vi "主程序.vi"() -> ()   [LabVIEW 2013]
doc: "该模板用于创建生产者／消费者模式的应用程序，以事件驱动的方式，生成队列中的项。如需通过响应事件实现代码的异步执行，同时不影响用户界面的响应速度，可考虑用该模式替代“用户界面事件处理器”模式。"
uses:
  <vilib>/Instr/_visa.llb/VISA Configure Serial Port (Instr).vi
panel:
  out "8位验证":string
  out "17位验证":string
  in  "参数保存":bool
  in  "执行次数":i32=3
  in  "减速（Max=65535）":i32=550 max=65535
  in  "加速（Max=65535）":i32=550 max=65535
  in  "行进距离（Max=16777214）":i32=25500 max=16777214
  out "低位":string
  out "高位":string
  out "运行速度（256-65535）":i32
  in  "位置控制模式":bool
  in  "模式选择":string(combo)="\u0000"
  in  "速度增减幅度":i32(ring)=1 items=["1"=1, "10"=10, "20"=20, "50"=50, "100"=100, "200"=200, "500"=500, "1000"=1000, "2000"=2000, "5000"=5000, "10000"=10000]
  in  "速度-":bool
  in  "速度+":bool
  in  "运行速度（256-65535）":i32=63500 min=256 max=65535
  in  "停止运行":bool
  in  "负向运行":bool
  in  "正向运行":bool
  in  "停止":bool
  in  "端口开关":bool
  in  "端口选择":refnum<visa-resource-name>
  # "步进电机控制系统"
  # "请关闭端口开关后再停止程序！"
  # "设置好相关参数后点击参数保存"
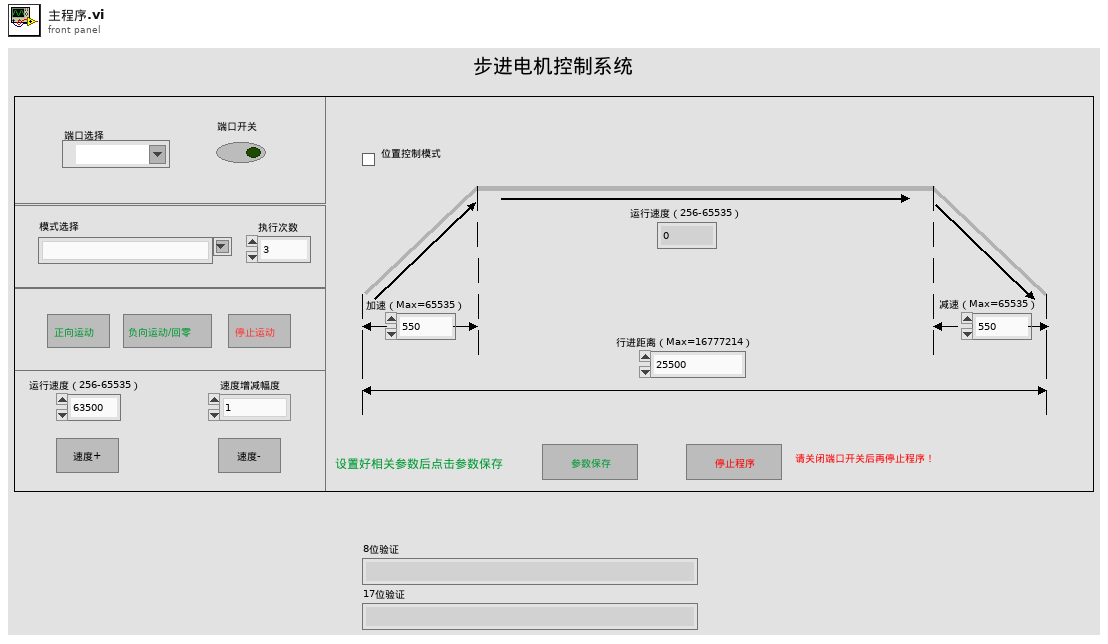
[diagram p1: front panel]
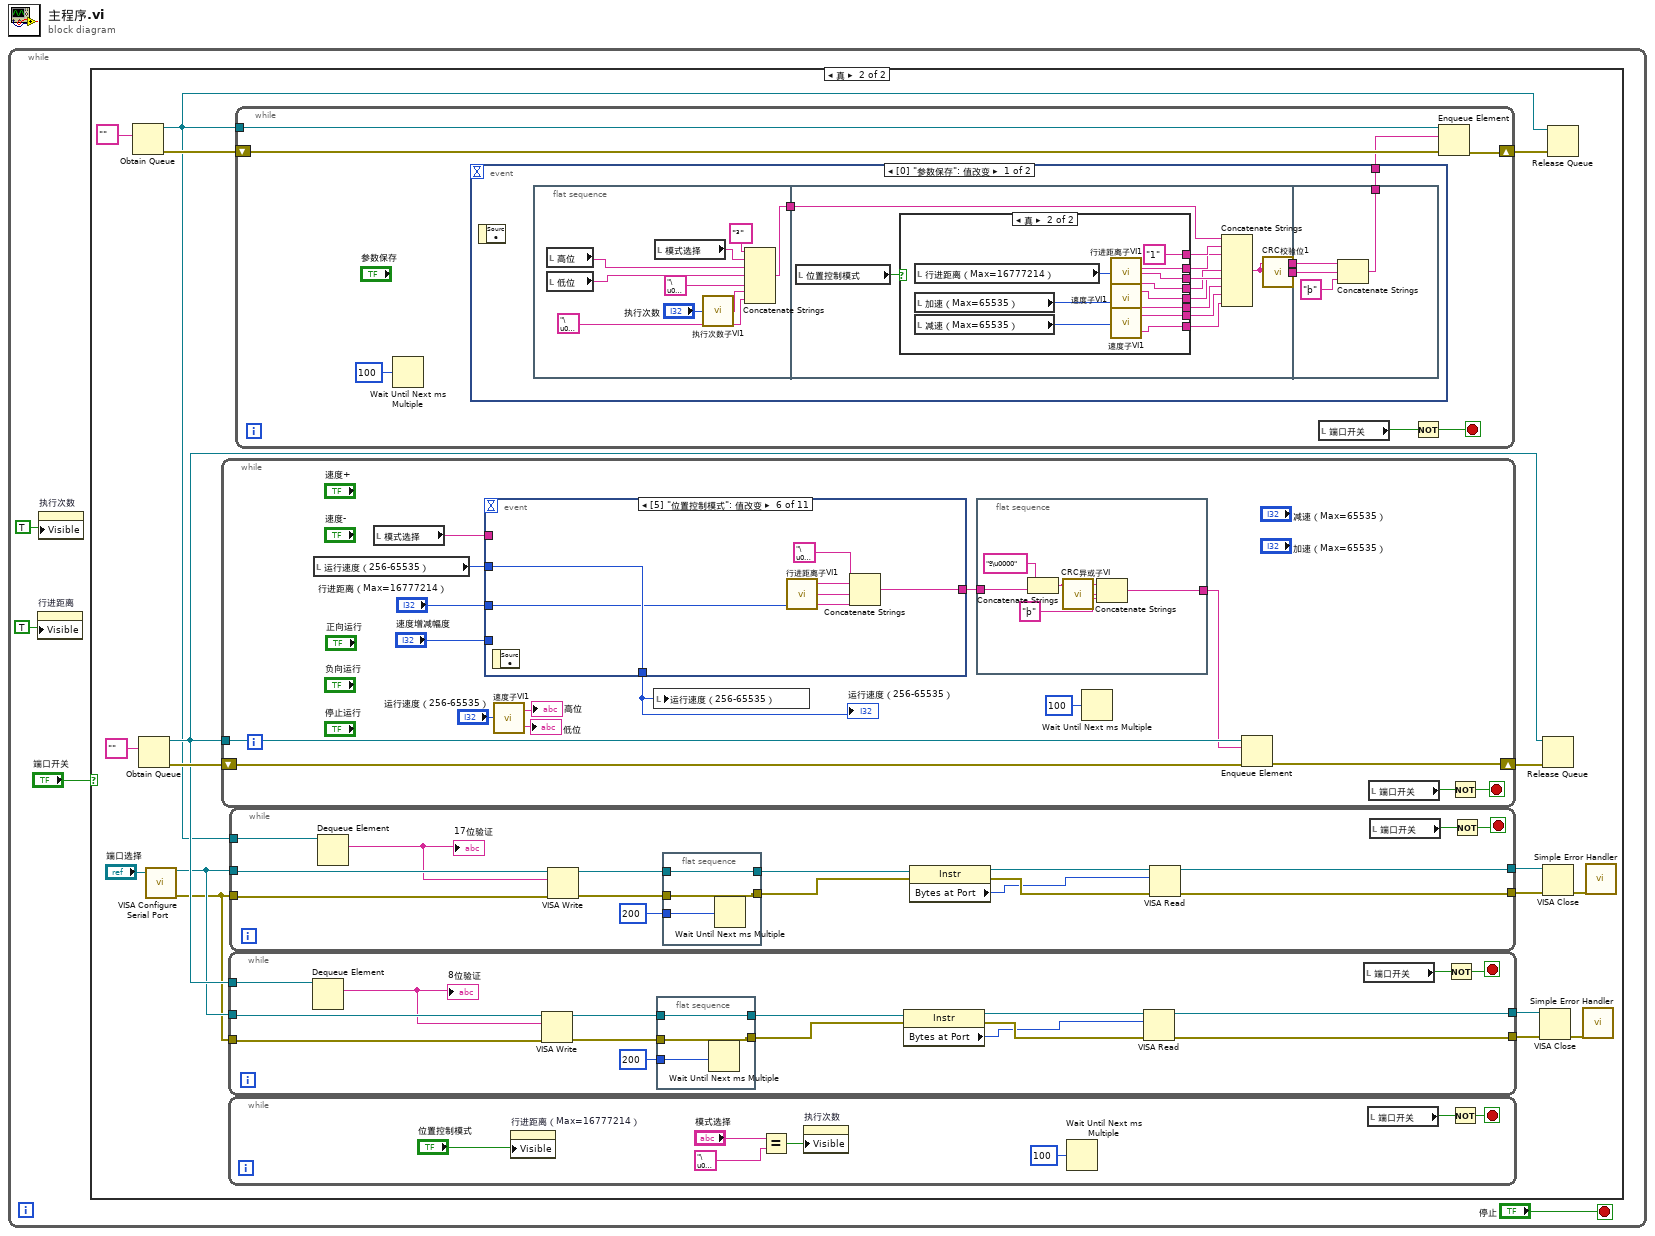
[diagram p0: block diagram]
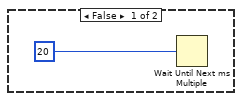
[diagram p2: hidden frame]
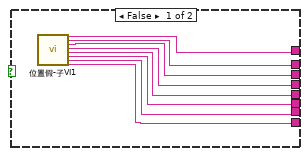
[diagram p3: hidden frame]
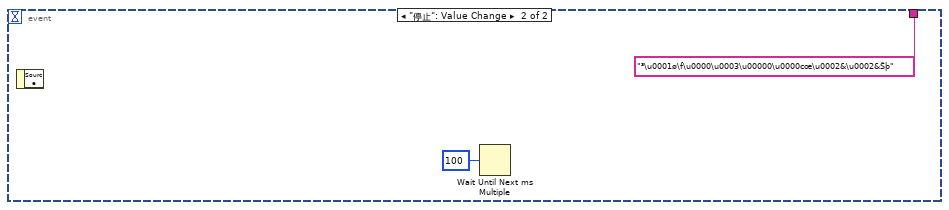
[diagram p4: hidden frame]
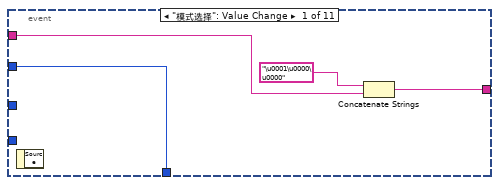
[diagram p5: hidden frame]
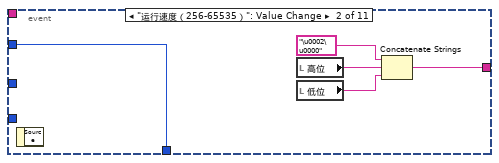
[diagram p6: hidden frame]
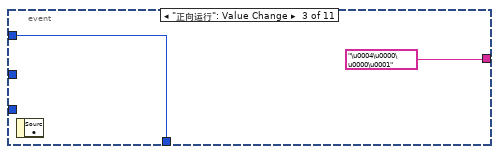
[diagram p7: hidden frame]
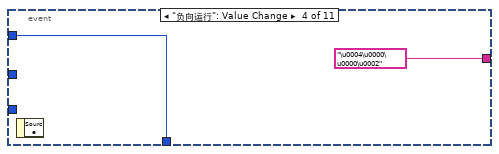
[diagram p8: hidden frame]
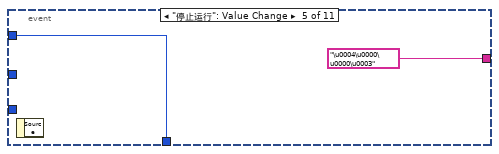
[diagram p9: hidden frame]
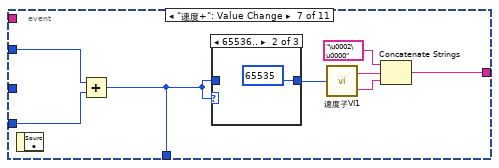
[diagram p10: hidden frame]
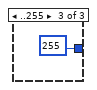
[diagram p12: hidden frame]
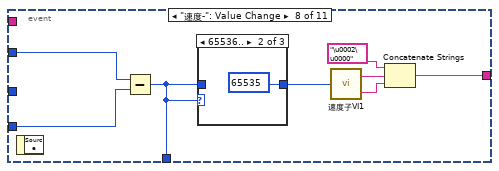
[diagram p13: hidden frame]
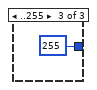
[diagram p15: hidden frame]
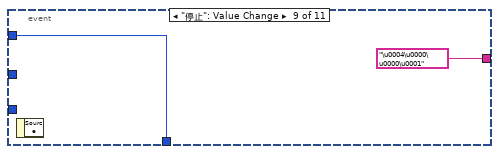
[diagram p16: hidden frame]
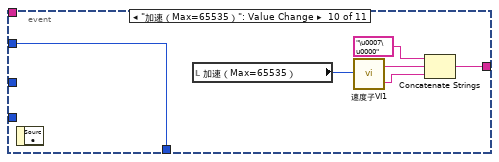
[diagram p17: hidden frame]
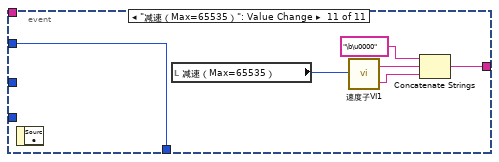
[diagram p18: hidden frame]
diagram:
  n1 = while {
    stop <- "停止" stop-if-true
    n2 = property on="行进距离" class="DigNum (严格)"("Visible"=TRUE) -> ()  [unwired: 2 in, 2 out]
    n3 = property on="执行次数" class="DigNum (严格)"("Visible"=TRUE) -> ()  [unwired: 2 in, 2 out]
    n4 = case shown="真" "端口开关" {
      frame False {
        n5 = Wait Until Next ms Multiple(millisecond multiple=u32 20 ("毫秒计时值")) -> ()  [unwired: 1 out]
      }
      frame True {
        n6 = Obtain Queue(element data type="") -> (queue out=w6:refnum<queue>, error out=w15:errorcluster)  [unwired: 4 in, 1 out]
        n7 = Obtain Queue(element data type="") -> (queue out=w12:refnum<queue>, error out=w22:errorcluster)  [unwired: 4 in, 1 out]
        n8 = call-poly "VISA Configure Serial Port"("VISA resource name"="端口选择") -> ("VISA resource name out"=w11:refnum<visa-resource-name>, "error out"=w10:errorcluster)  [unwired: 13 in]
        n9 = while {
          shift-right: [w139] -> w21
          shift-left: w22 -> [w140]
          tunnel: w12 -> [w138]
          stop <- w130 stop-if-true
          n10 = local read "运行速度（256-65535）"() -> (w129:i32)
          n11 = local read "模式选择"() -> (w126:string)
          n12 = event shown="[5] \"位置控制模式\": 值改变" {
            selector: _ -> [_ _ _ _ _ _ _ _ _ _ _]
            dyn-events: _ -> [_ _ _ _ _ _ _ _ _ _ _]
            timeout: _ -> [_ _ _ _ _ _ _ _ _ _ _]
            tunnel: [w149 w152 "\u0004\u0000\u0000\u0001" "\u0004\u0000\u0000\u0002" "\u0004\u0000\u0000\u0003" w164 w173 w184 "\u0004\u0000\u0000\u0001" w194 w200] -> w134
            tunnel: [w148 w151 w156 w158 w160 w163 w170 w182 w191 w193 w199] -> w133
            tunnel: w129 -> [w148 w151 w156 w158 w160 w163 w171 w181 w191 w193 w199]
            tunnel: "速度增减幅度" -> [_ _ _ _ _ _ w169 w180 _ _ _]
            tunnel: w126 -> [w147 _ _ _ _ _ _ _ _ _ _]
            tunnel: "行进距离（Max=16777214）" -> [_ _ _ _ _ w162 _ _ _ _ _]
            event "模式选择": Value Change {
              n13 = event-data() -> ()  [unwired: 1 in, 1 out]
              n14 = Concatenate Strings("\u0001\u0000\u0000", w147) -> (w149:string)
            }
            event "运行速度（256-65535）": Value Change {
              n15 = event-data() -> ()  [unwired: 1 in, 1 out]
              n16 = local read "高位"() -> (w154:string)
              n17 = local read "低位"() -> (w153:string)
              n18 = Concatenate Strings("\u0002\u0000", w154, w153) -> (w152:string)
            }
            event "正向运行": Value Change {
              n19 = event-data() -> ()  [unwired: 1 in, 1 out]
            }
            event "负向运行": Value Change {
              n20 = event-data() -> ()  [unwired: 1 in, 1 out]
            }
            event "停止运行": Value Change {
              n21 = event-data() -> ()  [unwired: 1 in, 1 out]
            }
            event "位置控制模式": Value Change {
              n22 = event-data() -> ()  [unwired: 1 in, 1 out]
              n23 = call "行进距离子VI1.vi"("脉冲输入端"=w162) -> ("行进脉冲总数高位"=w167:string, "行进脉冲总数中位"=w166:string, "行进脉冲总数低位"=w165:string)
              n24 = Concatenate Strings("\u0006", w167, w166, w165) -> (w164:string)
            }
            event "速度+": Value Change {
              n25 = event-data() -> ()  [unwired: 1 in, 1 out]
              n26 = Add(x=w171, y=w169) -> (x+y=w170:i32)
              n27 = case shown="65536.." w170 {
                tunnel: w170 -> [w177 _ _]
                tunnel: [w177 65535 255] -> w172
                frame 256..65535 {
                }
                frame 65536.. {
                }
                frame ..255 {
                }
              }
              n28 = call "速度子VI1.vi"("脉冲数"=w172) -> ("分频基数高位"=w175:string, "分频基数低位"=w174:string)
              n29 = Concatenate Strings("\u0002\u0000", w175, w174) -> (w173:string)
            }
            event "速度-": Value Change {
              n30 = event-data() -> ()  [unwired: 1 in, 1 out]
              n31 = Subtract(x=w181, y=w180) -> (x-y=w182:i32)
              n32 = case shown="65536.." w182 {
                tunnel: w182 -> [w188 _ _]
                tunnel: [w188 65535 255] -> w183
                frame 256..65535 {
                }
                frame 65536.. {
                }
                frame ..255 {
                }
              }
              n33 = call "速度子VI1.vi"("脉冲数"=w183) -> ("分频基数高位"=w186:string, "分频基数低位"=w185:string)
              n34 = Concatenate Strings("\u0002\u0000", w186, w185) -> (w184:string)
            }
            event "停止": Value Change {
              n35 = event-data() -> ()  [unwired: 1 in, 1 out]
            }
            event "加速（Max=65535）": Value Change {
              n36 = event-data() -> ()  [unwired: 1 in, 1 out]
              n37 = local read "加速（Max=65535）"() -> (w198:i32)
              n38 = call "速度子VI1.vi"("脉冲数"=w198) -> ("分频基数高位"=w196:string, "分频基数低位"=w195:string)
              n39 = Concatenate Strings("\u0007\u0000", w196, w195) -> (w194:string)
            }
            event "减速（Max=65535）": Value Change {
              n40 = event-data() -> ()  [unwired: 1 in, 1 out]
              n41 = local read "减速（Max=65535）"() -> (w204:i32)
              n42 = call "速度子VI1.vi"("脉冲数"=w204) -> ("分频基数高位"=w202:string, "分频基数低位"=w201:string)
              n43 = Concatenate Strings("\b\u0000", w202, w201) -> (w200:string)
            }
          }
          "运行速度（256-65535）" <- w133
          n44 = call "速度子VI1.vi"("脉冲数"="运行速度（256-65535）") -> ("分频基数高位"=→"高位":string, "分频基数低位"=→"低位":string)
          n45 = local write "运行速度（256-65535）"(w133) -> ()
          n46 = flat-sequence {
            tunnel: w134 -> [w145]
            tunnel: [w141] -> w127
            frame #0 {
              n47 = Concatenate Strings("º\u0000", w145) -> (w144:string)
              n48 = call "CRC异或子VI.vi"("输入"=w144) -> ("输出"=w143:string)
              n49 = Concatenate Strings(w144, w143, "þ") -> (w141:string)
            }
          }
          n50 = Wait Until Next ms Multiple(millisecond multiple=u32 100 ("毫秒倍数")) -> ()  [unwired: 1 out]
          n51 = Enqueue Element(queue=w138, element=w127, error in (no error)=w140) -> (error out=w139:errorcluster)  [unwired: 1 in, 2 out]
          n52 = local read "端口开关"() -> (w131:bool)
          n53 = Not(x=w131) -> (.not. x?=w130:bool)
        }
        n54 = while {
          tunnel: w10 -> [w26]
          tunnel: w11 -> [w27]
          tunnel: [w32] -> w7
          tunnel: [w31] -> w8
          tunnel: w12 -> [w28]
          stop <- w29 stop-if-true
          n55 = Dequeue Element(queue=w28) -> (element=w24:string)  [unwired: 2 in, 3 out]
          "8位验证" <- w24
          n56 = VISA Write(VISA resource name=w27, write buffer=w24, error in (no error)=w26) -> (VISA resource name out=w38:refnum<visa-resource-name>, error out=w37:errorcluster)  [unwired: 1 out]
          n57 = flat-sequence {
            tunnel: w38 -> [w41]
            tunnel: w37 -> [w40]
            tunnel: [w41] -> w36
            tunnel: [w40] -> w34
            tunnel: u32 200 ("等待时间（毫秒）") -> [w39]
            frame #0 {
              n58 = Wait Until Next ms Multiple(millisecond multiple=w39) -> ()  [unwired: 1 out]
            }
          }
          n59 = property class="Instr"(reference=w36, error in=w34) -> (reference out=w35:refnum<visa-resource-name>, error out=w33:errorcluster, "Bytes at Port"=w25:u32)
          n60 = VISA Read(VISA resource name=w35, byte count=w25, error in (no error)=w33) -> (VISA resource name out=w32:refnum<visa-resource-name>, error out=w31:errorcluster)  [unwired: 2 out]
          n61 = local read "端口开关"() -> (w30:bool)
          n62 = Not(x=w30) -> (.not. x?=w29:bool)
        }
        n63 = while {
          stop <- w103 stop-if-true
          n64 = property on="行进距离（Max=16777214）" class="DigNum (严格)"("Visible"="位置控制模式") -> ()  [unwired: 2 in, 2 out]
          n65 = Equal?(x="模式选择", y="\u0004") -> (x = y?=w99:bool)
          n66 = property on="执行次数" class="DigNum (严格)"("Visible"=w99) -> ()  [unwired: 2 in, 2 out]
          n67 = Wait Until Next ms Multiple(millisecond multiple=u32 100 ("等待时间（毫秒）")) -> ()  [unwired: 1 out]
          n68 = local read "端口开关"() -> (w104:bool)
          n69 = Not(x=w104) -> (.not. x?=w103:bool)
        }
        n70 = while {
          tunnel: w10 -> [w109]
          tunnel: w11 -> [w110]
          tunnel: [w115] -> w19
          tunnel: [w114] -> w18
          tunnel: w6 -> [w111]
          stop <- w112 stop-if-true
          n71 = Dequeue Element(queue=w111) -> (element=w107:string)  [unwired: 2 in, 3 out]
          "17位验证" <- w107
          n72 = VISA Write(VISA resource name=w110, write buffer=w107, error in (no error)=w109) -> (VISA resource name out=w121:refnum<visa-resource-name>, error out=w120:errorcluster)  [unwired: 1 out]
          n73 = flat-sequence {
            tunnel: w121 -> [w124]
            tunnel: w120 -> [w123]
            tunnel: [w124] -> w119
            tunnel: [w123] -> w117
            tunnel: u32 200 ("等待时间（毫秒）") -> [w122]
            frame #0 {
              n74 = Wait Until Next ms Multiple(millisecond multiple=w122) -> ()  [unwired: 1 out]
            }
          }
          n75 = property class="Instr"(reference=w119, error in=w117) -> (reference out=w118:refnum<visa-resource-name>, error out=w116:errorcluster, "Bytes at Port"=w108:u32)
          n76 = VISA Read(VISA resource name=w118, byte count=w108, error in (no error)=w116) -> (VISA resource name out=w115:refnum<visa-resource-name>, error out=w114:errorcluster)  [unwired: 2 out]
          n77 = local read "端口开关"() -> (w113:bool)
          n78 = Not(x=w113) -> (.not. x?=w112:bool)
        }
        n79 = while {
          tunnel: w6 -> [w46]
          shift-right: [w48] -> w14
          shift-left: w15 -> [w47]
          stop <- w43 stop-if-true
          n80 = Wait Until Next ms Multiple(millisecond multiple=u32 100 ("毫秒计时值")) -> ()  [unwired: 1 out]
          n81 = event shown="[0] \"参数保存\": 值改变" {
            selector: _ -> [_ _]
            dyn-events: _ -> [_ _]
            timeout: _ -> [_ _]
            tunnel: [w49 "³\u0001ø\f\u0000\u0003\u00000\u0000cœ\u0002&\u0002&Šþ"] -> w45
            event "参数保存": Value Change {
              n82 = event-data() -> ()  [unwired: 1 in, 1 out]
              n83 = flat-sequence {
                tunnel: [w57] -> w52
                tunnel: w52 -> [w65]
                tunnel: [w63] -> w51
                tunnel: [w62] -> w50
                tunnel: w51 -> [w95]
                tunnel: w50 -> [w94]
                tunnel: [w93] -> w49
                frame #0 {
                  n84 = local read "高位"() -> (w55:string)
                  n85 = local read "低位"() -> (w54:string)
                  n86 = local read "模式选择"() -> (w56:string)
                  n87 = call "执行次数子VI1.vi"("执行次数"="执行次数") -> ("HEX显示"=w59:string)
                  n88 = Concatenate Strings("³" ("字符串"), w56, w55, w54, "\u0000", w59, "\u0000" ("字符串")) -> (w57:string)
                }
                frame #1 {
                  n89 = local read "位置控制模式"() -> (w64:bool)
                  n90 = case shown="真" w64 {
                    tunnel: [w74 w92] -> w66
                    tunnel: [w75 w91] -> w67
                    tunnel: [w76 w90] -> w68
                    tunnel: [w77 w89] -> w69
                    tunnel: [w78 w88] -> w70
                    tunnel: [w79 w87] -> w71
                    tunnel: [w80 w86] -> w72
                    tunnel: [w81 "1"] -> w73
                    frame False {
                      n91 = call "位置假-子VI1.vi"() -> ("8"=w81:string, "9"=w80:string, "10"=w79:string, "11"=w78:string, "12"=w77:string, "13"=w76:string, "14"=w75:string, "15"=w74:string)  [unwired: 20 in]
                    }
                    frame True {
                      n92 = local read "行进距离（Max=16777214）"() -> (w84:i32)
                      n93 = local read "加速（Max=65535）"() -> (w83:i32)
                      n94 = local read "减速（Max=65535）"() -> (w82:i32)
                      n95 = call "行进距离子VI1.vi"("脉冲输入端"=w84) -> ("行进脉冲总数高位"=w86:string, "行进脉冲总数中位"=w87:string, "行进脉冲总数低位"=w88:string)
                      n96 = call "速度子VI1.vi"("脉冲数"=w83) -> ("分频基数高位"=w89:string, "分频基数低位"=w90:string)
                      n97 = call "速度子VI1.vi"("脉冲数"=w82) -> ("分频基数高位"=w91:string, "分频基数低位"=w92:string)
                    }
                  }
                  n98 = Concatenate Strings(w65, w73, w72, w71, w70, w69, w68, w67, w66) -> (w62:string)
                  n99 = call "CRC校验位1.vi"("输入端"=w62) -> ("CRC校验位"=w63:string)
                }
                frame #2 {
                  n100 = Concatenate Strings(w94, w95, "þ" ("字符串")) -> (w93:string)
                }
              }
            }
            event "停止": Value Change {
              n101 = event-data() -> ()  [unwired: 1 in, 1 out]
              n102 = Wait Until Next ms Multiple(millisecond multiple=u32 100 ("毫秒计时值")) -> ()  [unwired: 1 out]
            }
          }
          n103 = local read "端口开关"() -> (w44:bool)
          n104 = Not(x=w44) -> (.not. x?=w43:bool)
          n105 = Enqueue Element(queue=w46, element=w45, error in (no error)=w47) -> (error out=w48:errorcluster)  [unwired: 1 in, 2 out]
        }
        n106 = VISA Close(VISA resource name=w7, error in (no error)=w8) -> (error out=w9:errorcluster)
        n107 = Release Queue(queue=w12, error in (no error)=w21) -> ()  [unwired: 1 in, 3 out]
        n108 = VISA Close(VISA resource name=w19, error in (no error)=w18) -> (error out=w13:errorcluster)
        n109 = Release Queue(queue=w6, error in (no error)=w14) -> ()  [unwired: 1 in, 3 out]
        n110 = call <vilib>:"Simple Error Handler.vi"("error in (no error)"=w9) -> ()  [unwired: 4 in, 5 out]
        n111 = call <vilib>:"Simple Error Handler.vi"("error in (no error)"=w13) -> ()  [unwired: 4 in, 5 out]
      }
    }
  }
